vi "PPMS2_STD (SubVI).vi"(0 "Comments":string="Current source: 7/3\nVoltage sensing: 1/2, 4/2\nFreq. 0.745Hz", 5 "Experiment Folder Name":string="Sweep Vbg diff Field") -> (1 "Temperature (K)":dbl, 2 "appended path":path, 3 "filename":string, 4 "Numeric Control 2":dbl, 6 "String":string, 8 "Vbg":dbl, 10 "Field (Oe)":dbl, 12 "DC":dbl, 13 "Numeric Control":dbl, 14 "Position (Degree)":dbl)   [LabVIEW 2013]
uses:
  <userlib>/LevyLab/PPMS VI/SubVI/ITX_Global.vi
  PPMS Global.vi
  Lock-in Globals Multiple Inputs and Outputs.vi
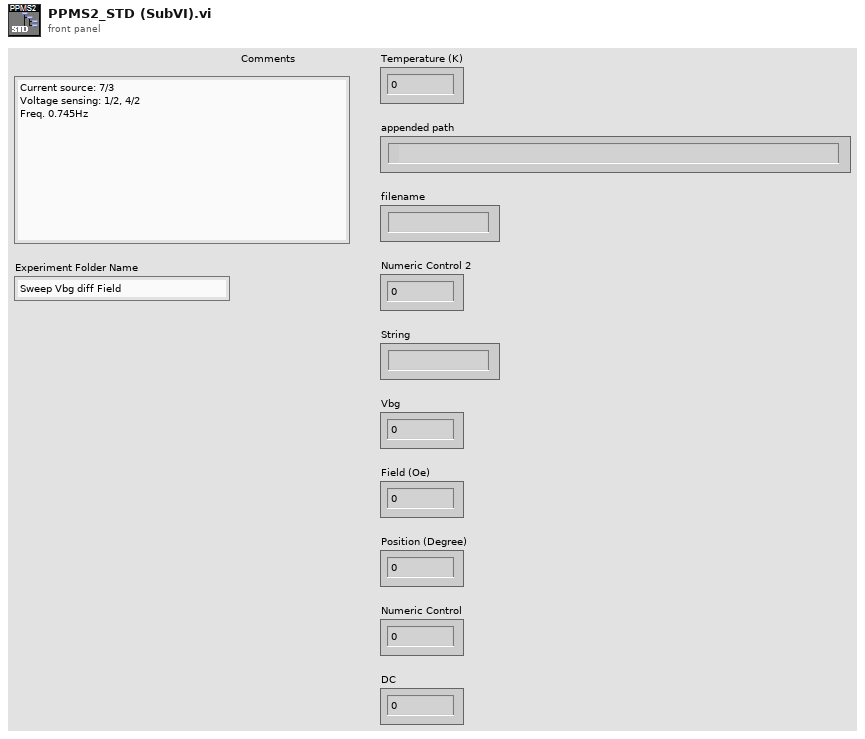
[diagram p1: front panel]
types:
  T1 = cluster{"Signal Type":enum16{"Sine Wave", "Triangle Wave", "Square Wave", "Sawtooth Wave"}, "DC":dbl, "Amplitude":dbl, "frequency":dbl, "Phase":dbl}[]
  T2 = cluster{"Signal Type":enum16{"Sine Wave", "Triangle Wave", "Square Wave", "Sawtooth Wave"}, "DC":dbl, "Amplitude":dbl, "frequency":dbl, "Phase":dbl}
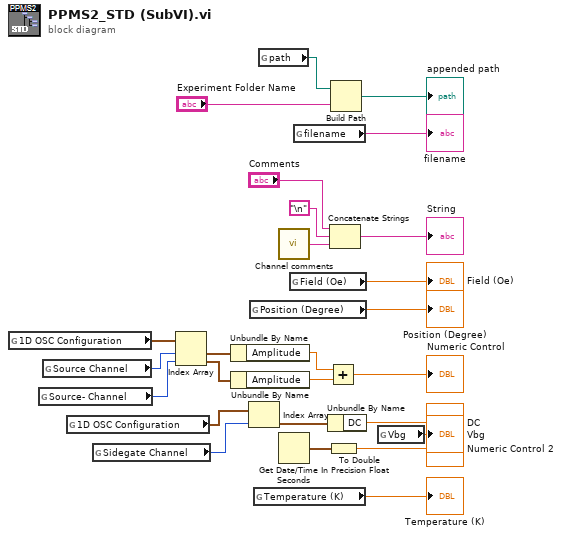
[diagram p0: block diagram]
diagram:
  n1 = global read "Lock-in Globals Multiple Inputs and Outputs.vi" "1D OSC Configuration"() -> (w15:T1)
  n2 = global read "Lock-in Globals Multiple Inputs and Outputs.vi" "Source- Channel"() -> (w19:i32)
  n3 = global read "Lock-in Globals Multiple Inputs and Outputs.vi" "Source Channel"() -> (w20:i32)
  n4 = global read "Lock-in Globals Multiple Inputs and Outputs.vi" "1D OSC Configuration"() -> (w23:T1)
  n5 = global read "Lock-in Globals Multiple Inputs and Outputs.vi" "Sidegate Channel"() -> (w24:i32)
  n6 = Index Array(array=w15, index #1=w20, index #2=w19) -> (element #1=w14:T2, element #2=w16:T2)
  n7 = Unbundle By Name(w14) -> ("Amplitude"=w17:dbl)
  n8 = Unbundle By Name(w16) -> ("Amplitude"=w18:dbl)
  n9 = Index Array(array=w23, index=w24) -> (element=w22:T2)
  n10 = global read "PPMS Global.vi" "Position (Degree)"() -> (→"Position (Degree)":dbl)
  n11 = global read "PPMS Global.vi" "Temperature (K)"() -> (→"Temperature (K)":dbl)
  n12 = global read "ITX_Global.vi" "path"() -> (w5:path)
  n13 = call "Channel comments.vi"() -> ("Comments on channels"=w3:string)  [unwired: 1 in]
  n14 = Get Date/Time In Seconds() -> (seconds since 1Jan1904=w9:timestamp)
  n15 = global read "PPMS Global.vi" "Field (Oe)"() -> (→"Field (Oe)":dbl)
  n16 = global read "ITX_Global.vi" "filename"() -> (→"filename":string)
  n17 = Add(x=w17, y=w18) -> (x+y=→"Numeric Control":dbl)
  n18 = Unbundle By Name(w22) -> ("DC"=→"DC":dbl)
  n19 = To Double Precision Float(number=w9) -> (double precision float=→"Numeric Control 2":dbl)
  n20 = Concatenate Strings("Comments", "\n", w3) -> (→"String":string)
  n21 = Build Path(base path=w5, name or relative path="Experiment Folder Name") -> (appended path=→"appended path":path)
  n22 = global read "Lock-in Globals Multiple Inputs and Outputs.vi" "Vbg"() -> (→"Vbg":dbl)
